vi "Pico_move_new.vi"(0 "Motor":i32, 1 "CmdLib Out":refnum<k24>, 2 "DeviceKey Out":string, 5 "Start Position":i32, 7 "Boolean 2":bool, 9 "Relative Steps":i32, 11 "Boolean":bool, 12 "error out":errorcluster, 13 "Device Address Out":i32) -> (4 "CmdLib Out":refnum<k24>, 6 "DeviceKey Out":string, 8 "Device Address Out":i32, 10 "error out 2":errorcluster)   [LabVIEW 2014]
uses:
  C:/Program Files/New Focus/New Focus Picomotor Application/Samples/CmdLib.dll
  Program Files/New Focus/New Focus Picomotor Application/Samples/CmdLib.dll
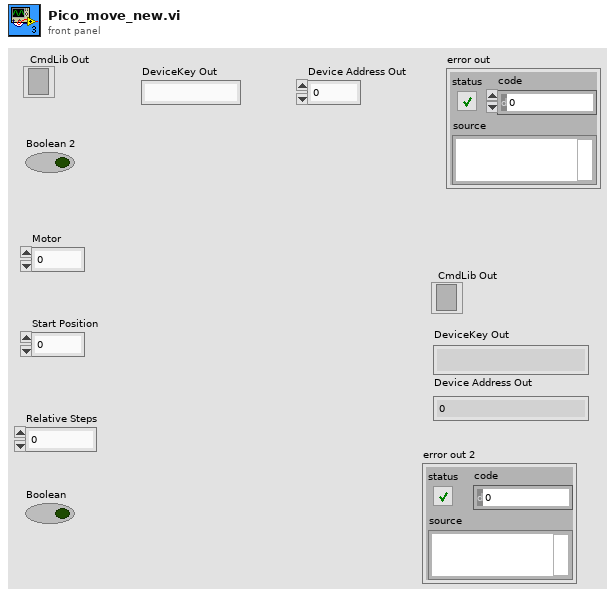
[diagram p1: front panel]
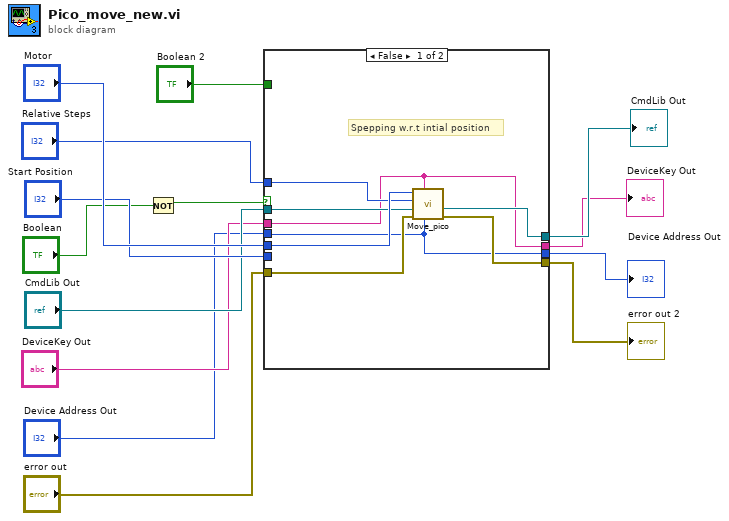
[diagram p0: block diagram]
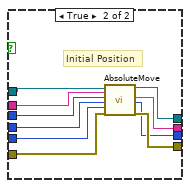
[diagram p3: hidden frame]
diagram:
  n1 = Not(x="Boolean") -> (.not. x?=w11:bool)
  n2 = case shown="False" w11 {
    tunnel: "CmdLib Out" -> [w20 w33]
    tunnel: "Device Address Out" -> [w15 w32]
    tunnel: "DeviceKey Out" -> [w16 w31]
    tunnel: "Motor" -> [w22 w30]
    tunnel: "Start Position" -> [_ w29]
    tunnel: "error out" -> [w19 w28]
    tunnel: [w18 w27] -> w1
    tunnel: [w16 w26] -> w5
    tunnel: [w15 w25] -> w3
    tunnel: "Relative Steps" -> [w21 _]
    tunnel: [w17 w24] -> w7
    tunnel: "Boolean 2" -> [_ w23]
    frame False {
      # "Spepping w.r.t intial position"
      n3 = call "Move_pico.vi"("Device Address In"=w15, "DeviceKey In"=w16, "error in (no error)"=w19, "CmdLib In"=w20, "Relative Steps"=w21, "Motor #"=w22) -> ("error out 2"=w18:errorcluster, "CmdLib Out"=w17:refnum<k24>)  [unwired: 4 in]
    }
    frame True {
      n4 = case shown="False" w23 {
        tunnel: w33 -> [w37 w47]
        tunnel: w32 -> [w35 w46]
        tunnel: w31 -> [w36 w45]
        tunnel: w30 -> [_ w44]
        tunnel: w29 -> [_ w43]
        tunnel: w28 -> [w34 w42]
        tunnel: [w34 w41] -> w27
        tunnel: [w36 w40] -> w26
        tunnel: [w35 w39] -> w25
        tunnel: [w37 w38] -> w24
        frame False {
        }
        frame True {
          # "Initial Position"
          n5 = call "AbsoluteMove.vi"("CmdLib In"=w47, "DeviceKey In"=w45, "Device Address In"=w46, "Motor"=w44, "Target Pos"=w43, "error in (no error)"=w42) -> ("CmdLib Out"=w38:refnum<k24>, "DeviceKey Out"=w40:string, "Device Address Out"=w39:i32, "error out"=w41:errorcluster)  [unwired: 10 in]
        }
      }
    }
  }
  "CmdLib Out" <- w7
  "DeviceKey Out" <- w5
  "Device Address Out" <- w3
  "error out 2" <- w1
